vi "Get Error.vi"(8 "error in (no error)":errorcluster, 11 "function return":u32) -> (0 "error out":errorcluster)   [LabVIEW 2023, in "PCAN API.lvlib"]
doc: "This VI creates errors from function return number."
uses:
  PCAN API.lvlib
  PCAN2023/PCAN2023.lvlib
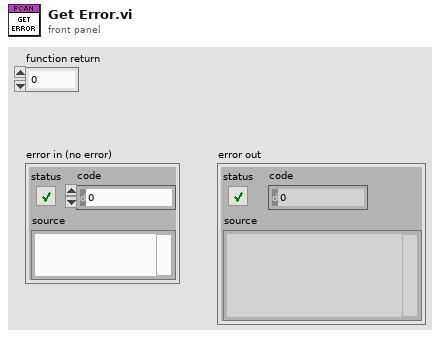
[diagram p1: front panel]
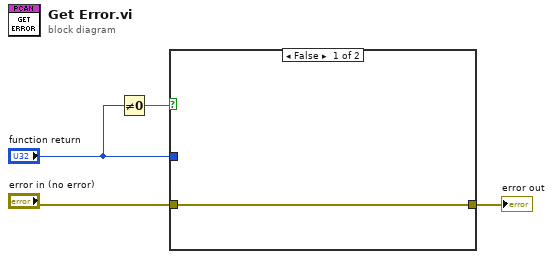
[diagram p0: block diagram]
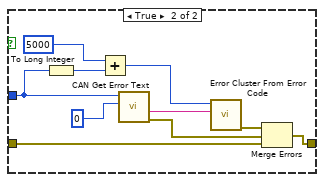
[diagram p2: hidden frame]
diagram:
  n1 = Not Equal To 0?(x="function return") -> (x != 0?=w1:bool)
  n2 = case shown="False" w1 {
    tunnel: "function return" -> [_ w12]
    tunnel: "error in (no error)" -> [w5 w7]
    tunnel: [w5 w6] -> w3
    frame False {
    }
    frame True {
      n3 = To Long Integer(number=w12) -> (32bit integer=w14:i32)
      n4 = Add(x=5000, y=w14) -> (x+y=w15:i32)
      n5 = call "CAN Get Error Text.vi"("Language"=u16 0, "Error"=w12) -> ("error out"=w8:errorcluster, "Buffer out"=w11:string)  [unwired: 7 in, 1 out]
      n6 = call <vilib>:"Error Cluster From Error Code.vi"("error message (\"\")"=w11, "error code (0)"=w15) -> ("error out"=w9:errorcluster)  [unwired: 7 in]
      n7 = Merge Errors(w9, w8, w7) -> (w6:errorcluster)
    }
  }
  "error out" <- w3
